vi "Get xwpfRef.vi"(8 "error in (no error)":errorcluster, 11 "xwpfReader in":refnum<class "xwpfReader.lvclass">) -> (0 "error out":errorcluster, 2 "xwpfRef":refnum<k24>, 3 "xwpfReader out":refnum<class "xwpfReader.lvclass">)   [LabVIEW 2017, in "xwpfReader.lvclass"]
uses:
  xwpfReader.lvclass
  C:/Users/Neo/Desktop/Dev_Tools_BR/LabVIEW_NPOI/src/lib/NPOI 2.1.1/NPOI.OOXML.dll
  lib/NPOI 2.1.1/NPOI.OOXML.dll
  xwpfReader.lvclass/xwpfReader.ctl
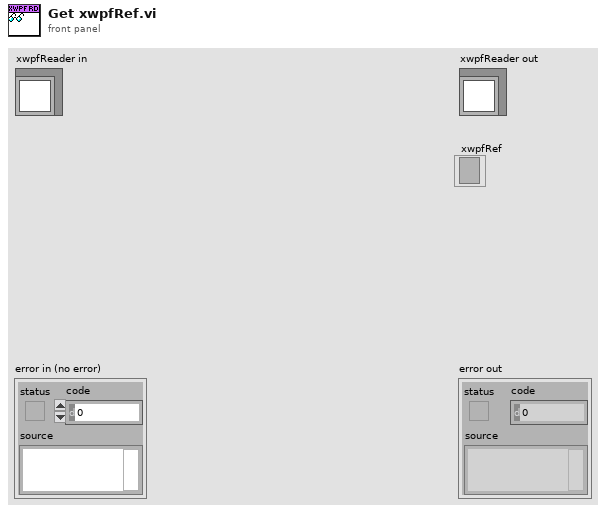
[diagram p1: front panel]
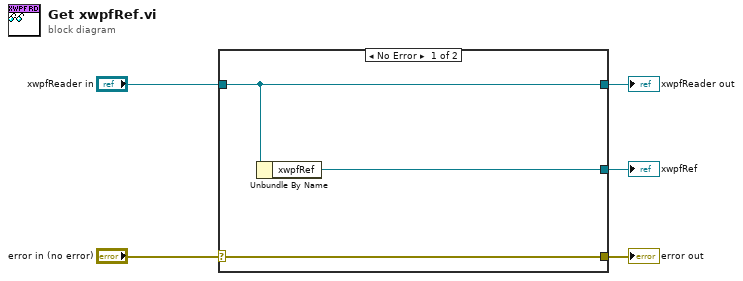
[diagram p0: block diagram]
diagram:
  n1 = case shown="No Error" "error in (no error)" {
    selector: "error in (no error)" -> [w8 w9]
    tunnel: [w8 w9] -> w4
    tunnel: [w7 w10] -> w2
    tunnel: "xwpfReader in" -> [w7 w10]
    tunnel: [w6 _] -> w1
    frame No Error {
      n2 = Unbundle By Name(w7) -> ("xwpfRef"=w6:refnum<k24>)
    }
    frame Error {
    }
  }
  "error out" <- w4
  "xwpfReader out" <- w2
  "xwpfRef" <- w1
